vi "160505-BM.vi"() -> ()   [LabVIEW 2013]
uses:
  Global_InitEndSync.vi
panel:
  in  "nVista":bool=TRUE
  out "Elapsed Time Text":string="0  00:05:14"
  in  "Duration on probe test (s)":u32=300
  in  "Top Button":bool
  in  "Gate Close / END Button":bool
  in  "Start Button":bool
  in  "ID":u8=1 min=1 max=21 step=1
  in  "Trial":u8=1 min=1 max=3 step=1
  in  "Phase":enum32{"Habituation", "Training", "Probe test"}(radio)=enum."Probe test"
  in  "Entry":enum8{"Lift", "Start-box", "Manual"}(ring)
  out "Mem usage (%)*":u8(slide)=23 caption="Slide 2" scale=0.0..100.0
  out "Save Path":path
  in  "Day":u8 max=20 step=1
  in  "Project Path":path
  in  "Frequency (Hz)":dbl=40.0
  out "General State":string="Finish"
  # "*メモリ使用量が 50% を超えたら，\nプログラムを再起動してください．"
  # "Click again, when the lift was stuck.\nControl up/down the lift from the buttons manually, \nif necessary."
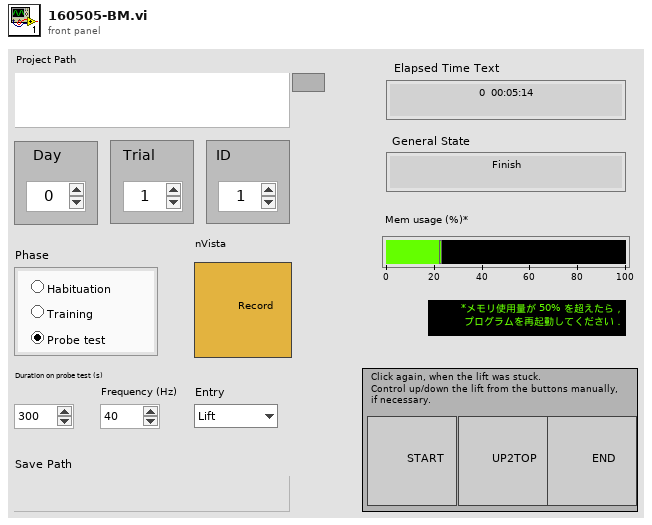
[diagram p1: front panel]
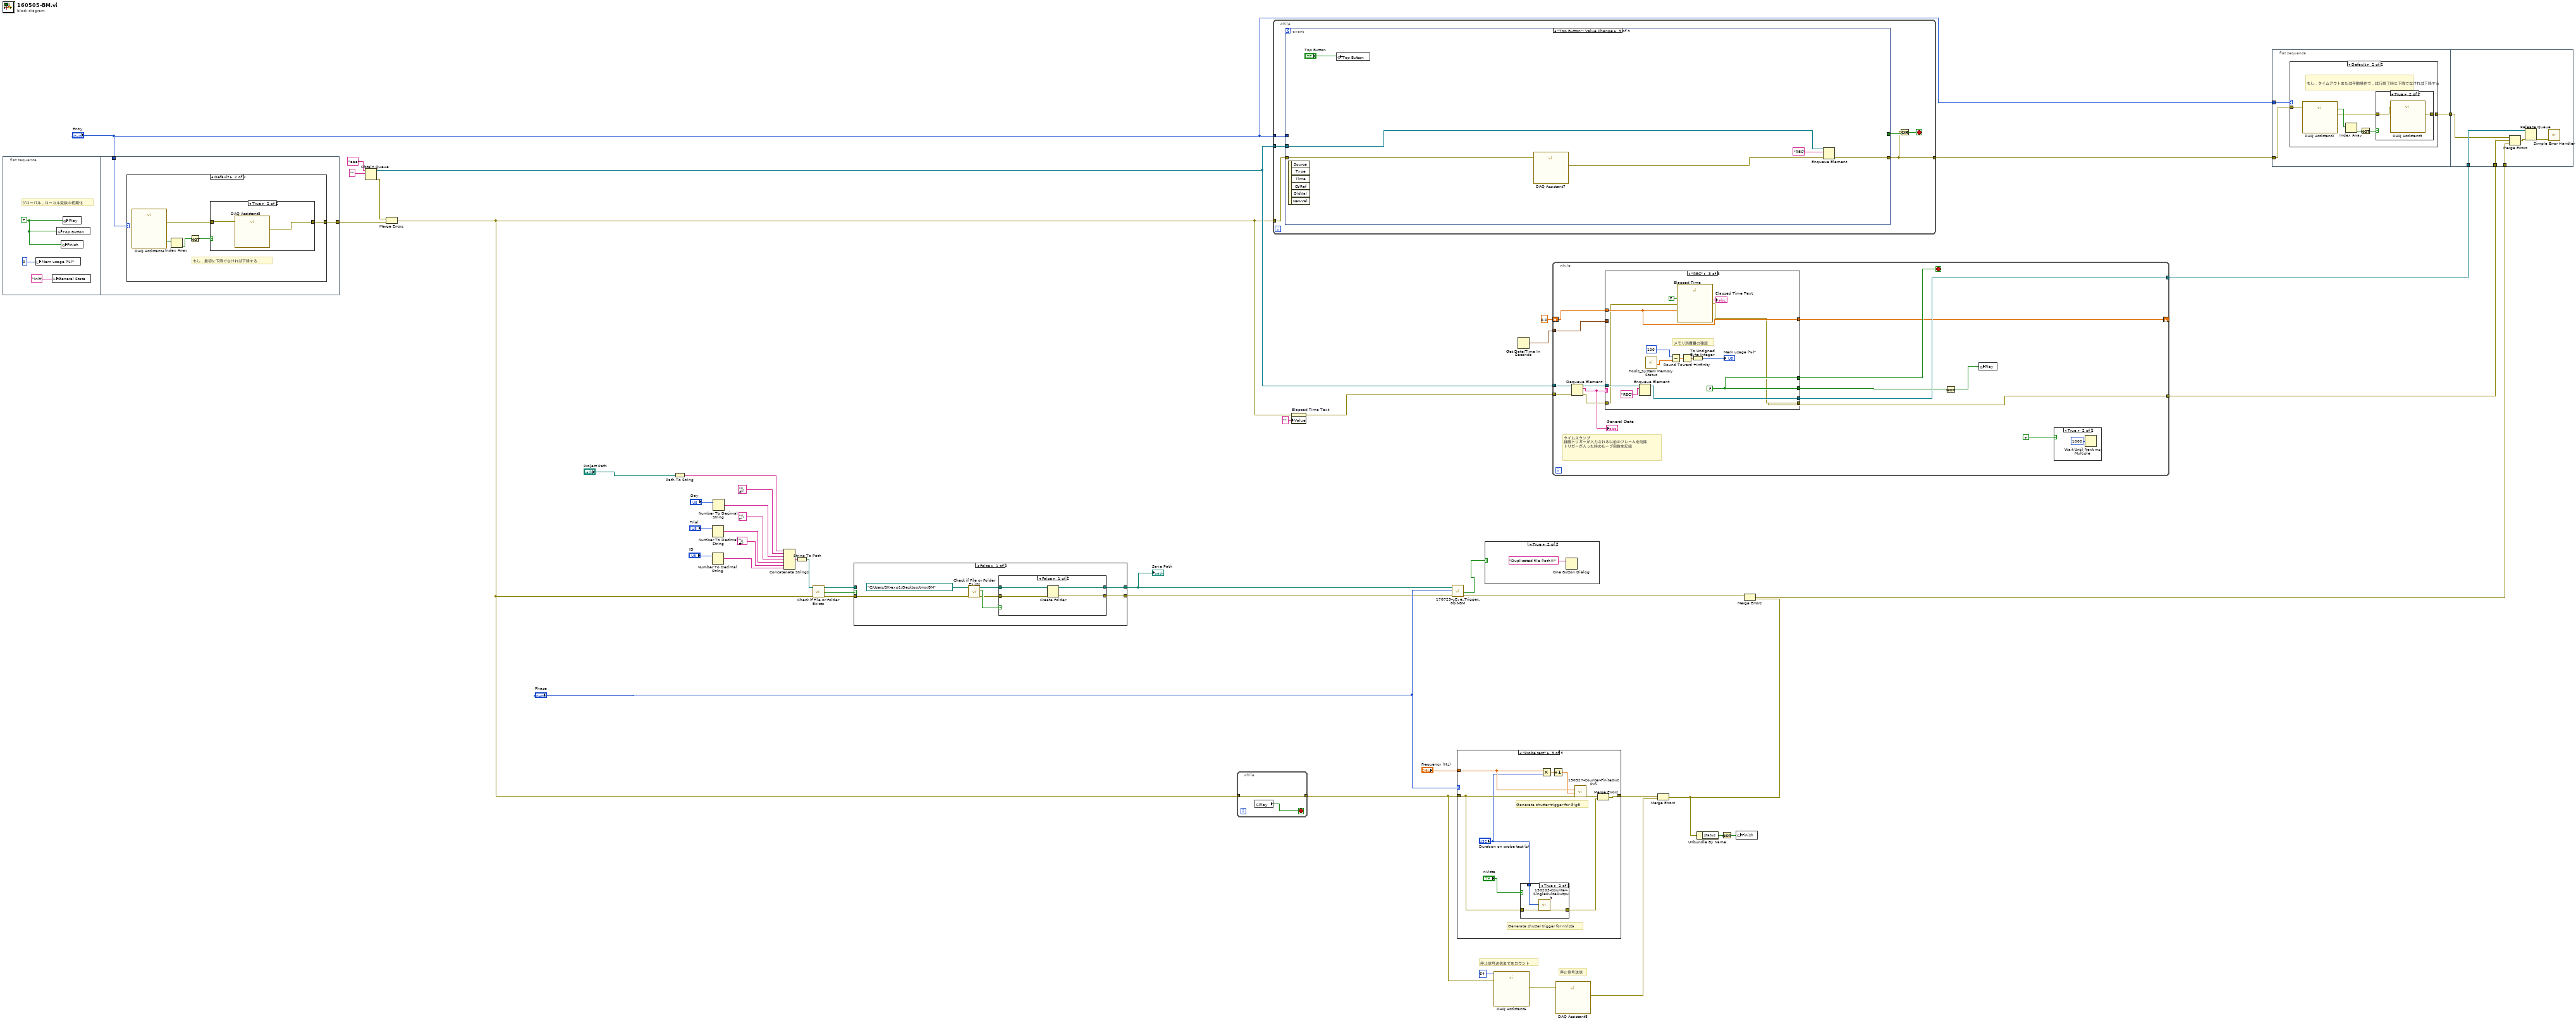
[diagram p0: block diagram]
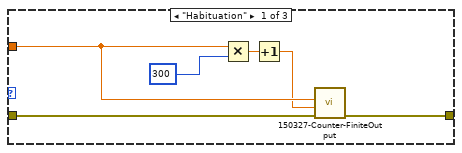
[diagram p3: hidden frame]
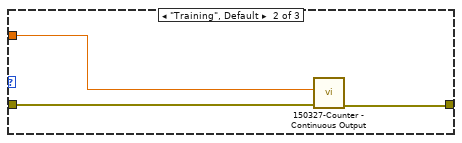
[diagram p4: hidden frame]
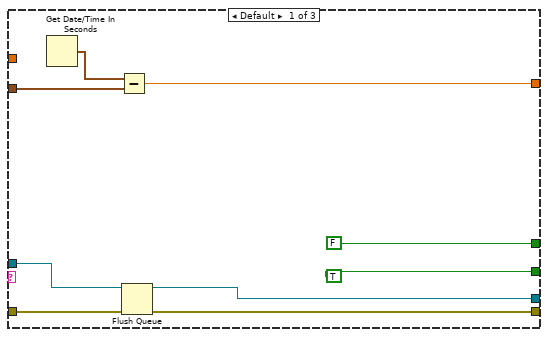
[diagram p9: hidden frame]
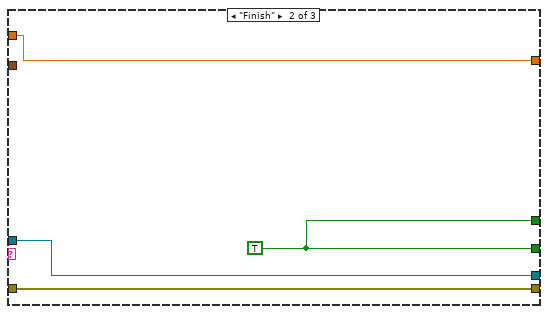
[diagram p10: hidden frame]
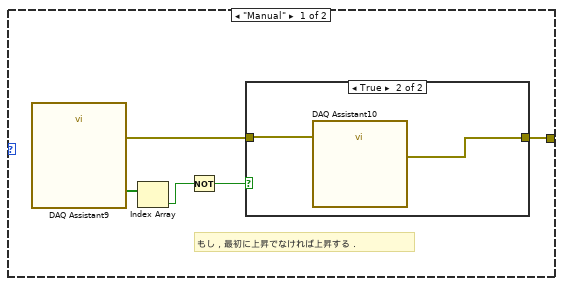
[diagram p11: hidden frame]
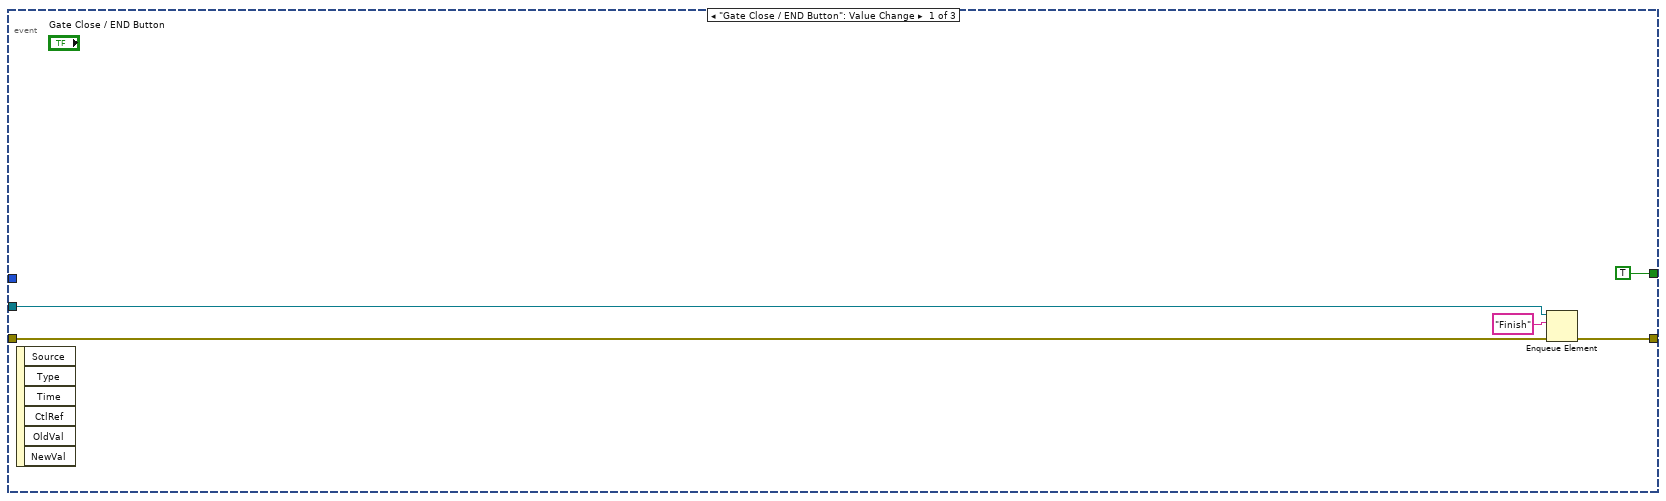
[diagram p16: hidden frame]
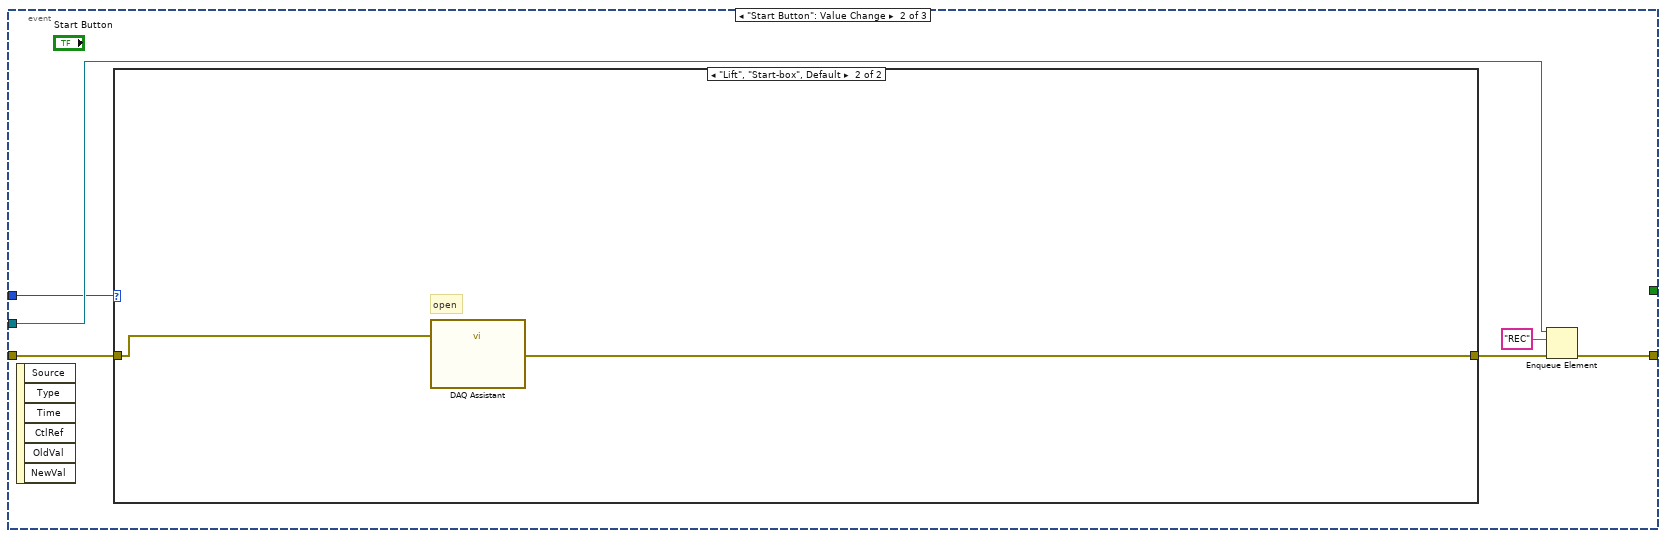
[diagram p17: hidden frame]
diagram:
  # "停止信号送信"
  # "停止信号送信までをカウント"
  n1 = flat-sequence {
    tunnel: [w51] -> w41
    tunnel: "Entry" -> [w50]
    frame #0 {
      w47 = FALSE
      # "グローバル，ローカル変数の初期化"
      n2 = local write "Mem usage (%)*"(0) -> ()
      n3 = local write "General State"("Init") -> ()
      n4 = global write "Global_InitEndSync.vi" "Top Button"(w47) -> ()
      n5 = global write "Global_InitEndSync.vi" "Finish"(w47) -> ()
      n6 = global write "Global_InitEndSync.vi" "Play"(w47) -> ()
    }
    frame #1 {
      n7 = case shown="Default" w50 {
        tunnel: [w52 w61] -> w51
        frame "Manual" {
          # "もし，最初に上昇でなければ上昇する．"
          n8 = call "DAQ Assistant9"() -> ("data"=w56:bool[], "error out"=w54:errorcluster)  [unwired: 17 in, 1 out]
          n9 = Index Array(array=w56) -> (element=w55:bool)  [unwired: 1 in]
          n10 = Not(x=w55) -> (.not. x?=w53:bool)
          n11 = case shown="True" w53 {
            tunnel: [w57 w59] -> w52
            tunnel: w54 -> [w57 w58]
            frame False {
            }
            frame True {
              n12 = call "DAQ Assistant10"("error in"=w58) -> ("error out"=w59:errorcluster)  [unwired: 17 in, 1 out]
            }
          }
        }
        frame Default {
          # "もし，最初に下降でなければ下降する．"
          n13 = call "DAQ Assistant4"() -> ("data"=w64:bool[], "error out"=w62:errorcluster)  [unwired: 17 in, 1 out]
          n14 = Index Array(array=w64) -> (element=w63:bool)  [unwired: 1 in]
          n15 = Not(x=w63) -> (.not. x?=w60:bool)
          n16 = case shown="True" w60 {
            tunnel: [w65 w67] -> w61
            tunnel: w62 -> [w65 w66]
            frame False {
            }
            frame True {
              n17 = call "DAQ Assistant5"("error in"=w66) -> ("error out"=w67:errorcluster)  [unwired: 17 in, 1 out]
            }
          }
        }
      }
    }
  }
  n18 = Obtain Queue(name (unnamed)="aaa", element data type="" ("element")) -> (queue out=w42:refnum<queue>, error out=w45:errorcluster)  [unwired: 3 in, 1 out]
  n19 = Merge Errors(w45, w41) -> (w9:errorcluster)
  n20 = Path To String(path="Project Path") -> (string=w16:string)
  n21 = Number To Decimal String(number="ID") -> (decimal integer string=w27:string)  [unwired: 1 in]
  n22 = Number To Decimal String(number="Trial") -> (decimal integer string=w29:string)  [unwired: 1 in]
  n23 = Number To Decimal String(number="Day") -> (decimal integer string=w32:string)  [unwired: 1 in]
  n24 = Concatenate Strings(w16, "\\d", w32, "\\t", w29, "\\#", w27) -> (w25:string)
  n25 = String To Path(string=w25) -> (path=w26:path)
  n26 = call <vilib>:"Check if File or Folder Exists.vi"("error in (no error)"=w9, "path"=w26) -> ("error out"=w22:errorcluster, "file or folder exists?"=w23:bool, "dup path"=w24:path)  [unwired: 7 in]
  n27 = case shown="False" w23 {
    tunnel: [w74 w82] -> w6
    tunnel: w24 -> [_ w82]
    tunnel: w22 -> [w72 w81]
    tunnel: [w68 w81] -> w4
    frame False {
      n28 = call <vilib>:"Check if File or Folder Exists.vi"("error in (no error)"=w72, "path"=path "C:/Users/SK-exp1/Desktop/tmp/BM" ("dup path")) -> ("error out"=w69:errorcluster, "file or folder exists?"=w71:bool, "dup path"=w70:path)  [unwired: 7 in]
      n29 = case shown="False" w71 {
        tunnel: [w78 w80] -> w74
        tunnel: w70 -> [w77 w80]
        tunnel: w69 -> [w76 w79]
        tunnel: [w75 w79] -> w68
        frame False {
          n30 = Create Folder(path (use dialog)=w77, error in=w76) -> (created path=w78:path, error out=w75:errorcluster)  [unwired: 1 in, 1 out]
        }
        frame True {
        }
      }
    }
    frame True {
    }
  }
  "Save Path" <- w6
  n31 = while {
    tunnel: w9 -> [w84]
    tunnel: [w84] -> w21
    stop <- w83 stop-if-true
    n32 = global read "Global_InitEndSync.vi" "Play"() -> (w83:bool)
  }
  n33 = while {
    tunnel: [w87] -> w46
    tunnel: w9 -> [w89]
    tunnel: w42 -> [w86]
    tunnel: "Entry" -> [w85]
    stop <- w88 stop-if-true
    n34 = event shown="[2] \"Top Button\": Value Change" {
      selector: _ -> [_ _ _]
      dyn-events: _ -> [_ _ _]
      timeout: _ -> [_ _ _]
      tunnel: [TRUE _ _] -> w90
      tunnel: [w92 w100 w108] -> w87
      tunnel: w89 -> [w93 w98 w106]
      tunnel: w86 -> [w94 w101 w109]
      tunnel: w85 -> [_ w96 _]
      event "Gate Close / END Button": Value Change {
        n35 = event-data() -> ()  [unwired: 1 in, 6 out]
        n36 = Enqueue Element(queue=w94, element="Finish", error in (no error)=w93) -> (error out=w92:errorcluster)  [unwired: 1 in, 2 out]
      }
      event "Start Button": Value Change {
        n37 = event-data() -> ()  [unwired: 1 in, 6 out]
        n38 = case shown="\"Lift\", \"Start-box\", Default" w96 {
          tunnel: w98 -> [w102 w103]
          tunnel: [w102 w104] -> w97
          frame "Manual" {
          }
          frame "Lift", "Start-box", Default {
            # "open"
            n39 = call "DAQ Assistant"("error in"=w103) -> ("error out"=w104:errorcluster)  [unwired: 17 in, 1 out]
          }
        }
        n40 = Enqueue Element(queue=w101, element="REC", error in (no error)=w97) -> (error out=w100:errorcluster)  [unwired: 1 in, 2 out]
      }
      event "Top Button": Value Change {
        n41 = event-data() -> ()  [unwired: 1 in, 6 out]
        n42 = global write "Global_InitEndSync.vi" "Top Button"("Top Button") -> ()
        n43 = call "DAQ Assistant7"("error in"=w106) -> ("error out"=w107:errorcluster)  [unwired: 17 in, 1 out]
        n44 = Enqueue Element(queue=w109, element="REC", error in (no error)=w107) -> (error out=w108:errorcluster)  [unwired: 1 in, 2 out]
      }
    }
    n45 = Or(x=w87, y=w90) -> (x .or. y?=w88:bool)
  }
  n46 = property on="Elapsed Time Text" class="Str"(error in=w9, "Value"="" ("Elapsed Time Text")) -> (error out=w8:errorcluster)  [unwired: 1 in, 1 out]
  n47 = call "170729-uEye_Trigger_8bit-BM.vi"("error in"=w4, "Phase"="Phase", "Save Path"=w6) -> ("error out"=w3:errorcluster, "DupFiles"=w2:bool)  [unwired: 5 in]
  n48 = case shown="\"Probe test\"" "Phase" {
    tunnel: w21 -> [w116 w118 w124]
    tunnel: [w115 w117 w123] -> w20
    tunnel: "Frequency (Hz)" -> [w114 w119 w126]
    frame "Habituation" {
      n49 = Multiply(x=w114, y=300) -> (x*y=w112:dbl)
      n50 = Increment(x=w112) -> (x+1=w113:dbl)
      n51 = call "150327-Counter-FiniteOutput.vi"("error in"=w116, "Number of Pulses"=w113, "Frequency"=w114) -> ("error out 2"=w115:errorcluster)  [unwired: 8 in]
    }
    frame "Training", Default {
      n52 = call "150327-Counter - Continuous Output.vi"("error in"=w118, "Frequency"=w119) -> ("error out 2"=w117:errorcluster)  [unwired: 9 in]
    }
    frame "Probe test" {
      # "Generate shutter trigger for nVista"
      # "Generate shutter trigger for GigE"
      n53 = case shown="True" "nVista" {
        tunnel: "Duration on probe test (s)" -> [_ w132]
        tunnel: w124 -> [w129 w131]
        tunnel: [w129 w130] -> w122
        frame False {
        }
        frame True {
          n54 = call "150203-Counter-SinglePulseOutput.vi"("error in"=w131, "Pulse Duration"=w132) -> ("error out 2"=w130:errorcluster)  [unwired: 9 in]
        }
      }
      n55 = Multiply(x=w126, y="Duration on probe test (s)") -> (x*y=w127:dbl)
      n56 = Increment(x=w127) -> (x+1=w128:dbl)
      n57 = call "150327-Counter-FiniteOutput.vi"("error in"=w124, "Number of Pulses"=w128, "Frequency"=w126) -> ("error out 2"=w125:errorcluster)  [unwired: 8 in]
      n58 = Merge Errors(w125, w122) -> (w123:errorcluster)
    }
  }
  n59 = case shown="True" w2 {
    frame False {
    }
    frame True {
      n60 = One Button Dialog(message="Duplicated file Path!!!" ("error source (\" \")")) -> ()  [unwired: 1 in, 1 out]
    }
  }
  n61 = call "DAQ Assistant6"("number of samples"=64, "error in"=w21) -> ("error out"=w12:errorcluster)  [unwired: 16 in, 1 out]
  n62 = Get Date/Time In Seconds() -> (seconds since 1Jan1904=w11:timestamp)
  n63 = while {
    tunnel: w42 -> [w147]
    tunnel: [w142] -> w38
    tunnel: w8 -> [w146]
    tunnel: [w139] -> w37
    tunnel: w11 -> [w136]
    shift-right: [w135] -> _
    shift-left: 0.0 -> [w134]
    stop <- w141 stop-if-true
    # "タイムスタンプ\n録画トリガーが入力される以前のフレームを削除\nトリガーが入った時のループ回数を記録"
    n64 = Dequeue Element(queue=w147, error in (no error)=w146) -> (queue out=w144:refnum<queue>, element=w143:string, error out=w145:errorcluster)  [unwired: 1 in, 1 out]
    "General State" <- w143
    n65 = case shown="\"REC\"" w143 {
      tunnel: [TRUE w159 w172] -> w138
      tunnel: w145 -> [w154 w160 w163]
      tunnel: [w153 w160 w162] -> w139
      tunnel: w144 -> [w156 w161 w175]
      tunnel: [w155 w161 w174] -> w142
      tunnel: [FALSE w159 w172] -> w141
      tunnel: w136 -> [w150 _ _]
      tunnel: [w149 w158 w164] -> w135
      tunnel: w134 -> [_ w158 w164]
      frame Default {
        n66 = Get Date/Time In Seconds() -> (seconds since 1Jan1904=w151:timestamp)
        n67 = Subtract(x=w151, y=w150) -> (x-y=w149:dbl)
        n68 = Flush Queue(queue=w156, error in (no error)=w154) -> (queue out=w155:refnum<queue>, error out=w153:errorcluster)  [unwired: 1 out]
      }
      frame "Finish" {
        w159 = TRUE
      }
      frame "REC" {
        w172 = FALSE
        # "メモリ消費量の確認"
        n69 = Enqueue Element(queue=w175, element="REC") -> (queue out=w174:refnum<queue>)  [unwired: 2 in, 2 out]
        n70 = call "Tools_System Memory Status.vi"() -> ("Free memory (%)"=w167:dbl)  [unwired: 8 in, 3 out]
        n71 = Subtract(x=100, y=w167) -> (x-y=w169:dbl)
        n72 = call "Elapsed Time"("Auto Reset"=FALSE, "error in (no error)"=w163, "Set Start Time (s)"=w164) -> ("Elapsed Time Text"=→"Elapsed Time Text":string, "error out"=w162:errorcluster)  [unwired: 9 in, 6 out]
        n73 = Round Toward +Infinity(x=w169) -> (ceil(x): smallest int >= x=w170:dbl)
        n74 = To Unsigned Byte Integer(number=w170) -> (unsigned 8bit integer=→"Mem usage (%)*":u8)
      }
    }
    n75 = Not(x=w138) -> (.not. x?=w137:bool)
    n76 = global write "Global_InitEndSync.vi" "Play"(w137) -> ()
    n77 = case shown="True" TRUE {
      frame False {
      }
      frame True {
        n78 = Wait Until Next ms Multiple(millisecond multiple=u32 1000) -> ()  [unwired: 1 out]
      }
    }
  }
  n79 = call "DAQ Assistant8"("error in"=w12) -> ("error out"=w19:errorcluster)  [unwired: 17 in, 1 out]
  n80 = Merge Errors(w20, w19) -> (w40:errorcluster)
  n81 = Unbundle By Name(w40) -> ("status"=w18:bool)
  n82 = Not(x=w18) -> (.not. x?=w17:bool)
  n83 = global write "Global_InitEndSync.vi" "Finish"(w17) -> ()
  n84 = Merge Errors(w3, w40) -> (w36:errorcluster)
  n85 = flat-sequence {
    tunnel: w46 -> [w176]
    tunnel: [w178] -> w39
    tunnel: "Entry" -> [w177]
    tunnel: w39 -> [w189]
    tunnel: w38 -> [w193]
    tunnel: w37 -> [w191]
    tunnel: w36 -> [w192]
    frame #0 {
      n86 = case shown="Default" w177 {
        tunnel: [w179 w185] -> w178
        tunnel: w176 -> [w179 w180]
        frame "Manual" {
        }
        frame Default {
          # "もし，タイムアウトまたは手動操作で，試行終了時に下降でなければ下降する"
          n87 = call "DAQ Assistant2"("error in"=w180) -> ("data"=w184:bool[], "error out"=w183:errorcluster)  [unwired: 16 in, 1 out]
          n88 = Index Array(array=w184) -> (element=w182:bool)  [unwired: 1 in]
          n89 = Not(x=w182) -> (.not. x?=w181:bool)
          n90 = case shown="True" w181 {
            tunnel: [w186 w188] -> w185
            tunnel: w183 -> [w186 w187]
            frame False {
            }
            frame True {
              n91 = call "DAQ Assistant3"("error in"=w187) -> ("error out"=w188:errorcluster)  [unwired: 17 in, 1 out]
            }
          }
        }
      }
    }
    frame #1 {
      n92 = Merge Errors(w189, w191, w192) -> (w194:errorcluster)
      n93 = Release Queue(queue=w193, error in (no error)=w194) -> (error out=w190:errorcluster)  [unwired: 1 in, 2 out]
      n94 = call <vilib>:"Simple Error Handler.vi"("error in (no error)"=w190) -> ()  [unwired: 4 in, 5 out]
    }
  }
